vi "Read Children.vi"(8 "Error In":errorcluster, 11 "Non-Terminal In":refnum<class "NonTerminal.lvclass">) -> (0 "Error Out":errorcluster, 2 "Children":refnum<class "Node.lvclass">[](array[class]), 3 "Non-Terminal Out":refnum<class "NonTerminal.lvclass">)   [LabVIEW 2018, in "Toolkit.lvlib" / "Nodes.lvlib" / "NonTerminal.lvclass"]
doc: "Gets all of the children nodes of this parent node. This does not recursively desend down children Non-Terminal nodes.\n\n<B>Non-Terminal In/Out</B> - Represents a node in an Abstract Syntax Tree (AST) of a parsed Mustache template that can have one or more children nodes.\n\n<B>Children</B> - All of the children of this parent, non-terminal node."
uses:
  NonTerminal.lvclass
  Node/Node.lvclass
  NonTerminal.lvclass/NonTerminal.ctl
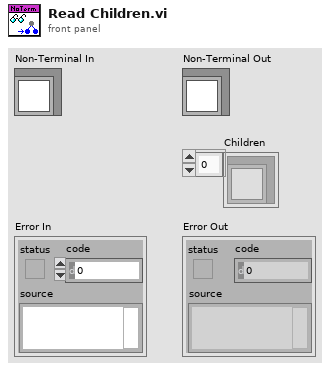
[diagram p1: front panel]
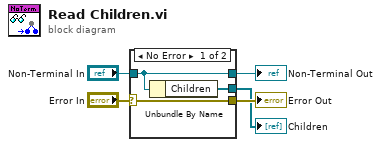
[diagram p0: block diagram]
diagram:
  n1 = case shown="No Error" "Error In" {
    selector: "Error In" -> [w8 w10]
    tunnel: [w8 w10] -> w4
    tunnel: [w7 w9] -> w2
    tunnel: "Non-Terminal In" -> [w7 w9]
    tunnel: [w6 _] -> w1
    frame No Error {
      n2 = Unbundle By Name(w7) -> ("Children"=w6:refnum<class "Node.lvclass">[])
    }
    frame Error {
    }
  }
  "Error Out" <- w4
  "Non-Terminal Out" <- w2
  "Children" <- w1
